vi "EtherNet_IP_CIP Demo.vi"() -> ()   [LabVIEW 2020, in "EtherNet_IP_CIP_Lib.lvlib"]
uses:
  EtherNet_IP_CIP_Lib.lvlib
panel:
  in  "CONTROL/TIMER/COUNTER":T1
  in  "REAL Array":sgl[](array[numeric])
  in  "DINT Array":u32[](array[numeric])
  in  "INT Array":u16[](array[numeric])
  in  "SINT Array":u8[](array[numeric])
  in  "BOOL Array":bool[](array[boolean])
  in  "BOOL Data":bool
  in  "Datatype":T2(ring)=enum."DINT"
  in  "Tag Name":string="EIPTXT01"
  in  "EtherNet/IP Device Address":string="192.168.1.214"
  out "REAL Array":sgl[](array[numeric])
  out "DINT Array":u32[](array[numeric]) format="%x"
  out "INT Array":u16[](array[numeric])
  out "SINT Array":u8[](array[numeric])
  out "CONTROL/TIMER/COUNTER":T1
  out "Datatype":T2(ring)
  out "BOOL Array":bool[](array[boolean])
  out "BOOL":bool
  out "Status":T3(ring)
  in  "Enter Tag Name":string="EIPTXT01"
  in  "No of Elements":u8
  out "Data Error":bool
  out "ms for Each Scan":u32
  out "error out":errorcluster
  in  "Exit":bool
  # "Write tag"
  # "Read Tag"
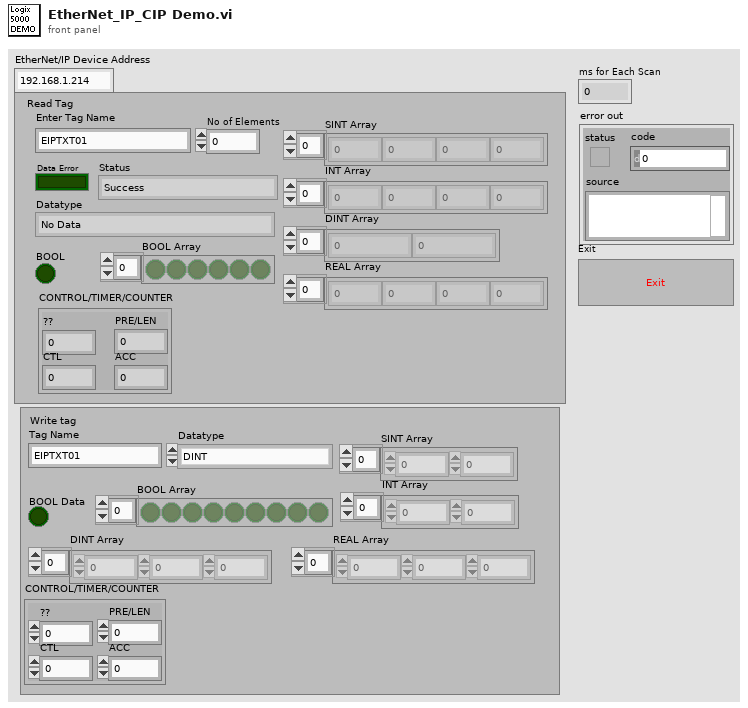
[diagram p1: front panel]
types:
  T1 = cluster{"??":u16, "CTL":u32, "PRE/LEN":u32, "ACC":u32}
  T2 = enum16{"No Data", "BOOL", "BIT Array", "SINT", "INT", "DINT", "REAL", "TIMER/CONTROL/COUNTER"}
  T3 = enum16{"Success", "Unknown Error", "Bad Symbolic Representation", "Item Not Found", "Partial Read", "Error Processing Attribute", "Incorrect/Insufficient Param", "Insufficient Attribute", "Bad Symbolic Length", "Out Of Bound", "Type Mismatch", "Offset Out Of Bound"}
  T4 = cluster{"TCP Connection":refnum<k5>, "Session":u8[], "EtherNet/IP Device Address":string}
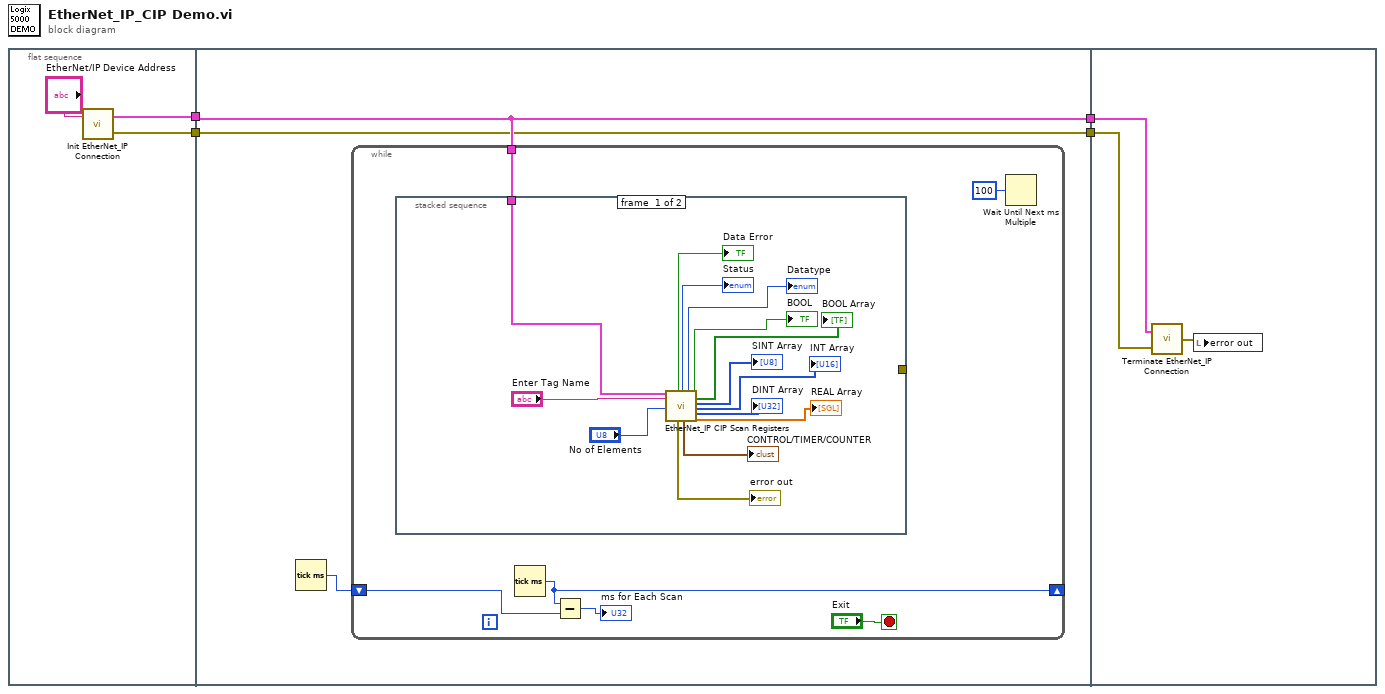
[diagram p0: block diagram]
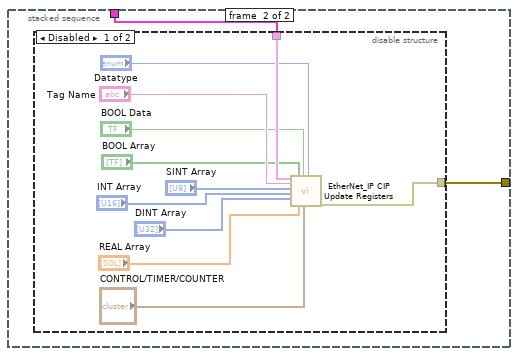
[diagram p2: hidden frame]
diagram:
  n1 = flat-sequence {
    tunnel: [w6] -> w4
    tunnel: [w5] -> w3
    tunnel: w4 -> [w10]
    tunnel: w3 -> [w8]
    tunnel: [w10] -> w2
    tunnel: [w8] -> w1
    tunnel: w2 -> [w46]
    tunnel: w1 -> [w45]
    frame #0 {
      n2 = call "Init EtherNet_IP Connection.vi"("EtherNet/IP Device Address"="EtherNet/IP Device Address") -> ("error out"=w5:errorcluster, "Connection Cluster"=w6:T4)  [unwired: 1 in]
    }
    frame #1 {
      n3 = Tick Count (ms)() -> (millisecond timer value=w9:u32)
      n4 = while {
        tunnel: w10 -> [w12]
        shift-right: [w15] -> _
        shift-left: w9 -> [w14]
        stop <- "Exit" stop-if-true
        n5 = stacked-sequence {
          tunnel: w12 -> [w29 w31]
          tunnel: [_ w32] -> _
          frame #0 {
            n6 = call "EtherNet_IP CIP Scan Registers.vi"("Connection Cluster"=w29, "Tag"="Enter Tag Name", "No of Elements"="No of Elements") -> ("Data Error"=→"Data Error":bool, "error out"=→"error out":errorcluster, "Status"=→"Status":T3, "CONTROL/TIMER/COUNTER"=→"CONTROL/TIMER/COUNTER":T1, "Datatype"=→"Datatype":T2, "BOOL"=→"BOOL":bool, "BOOL Array"=→"BOOL Array":bool[], "SINT Array"=→"SINT Array":u8[], "INT Array"=→"INT Array":u16[], "DINT Array"=→"DINT Array":u32[], "REAL Array"=→"REAL Array":sgl[])  [unwired: 5 in, 1 out]
          }
          frame #1 {
            n7 = disable-structure shown="Disabled" {
              disable-tunnel: [w42 _] -> w32
              disable-tunnel: w31 -> [w41 _]
              frame Disabled {
                n8 = call "EtherNet_IP CIP Update Registers.vi"("Connection Cluster"=w41, "Tag"="Tag Name", "SINT Array"="SINT Array", "INT Array"="INT Array", "DINT Array"="DINT Array", "BOOL Array"="BOOL Array", "REAL Array"="REAL Array", "BOOL"="BOOL Data", "CONTROL/TIMER/COUNTER"="CONTROL/TIMER/COUNTER", "Datatype"="Datatype") -> ("error out"=w42:errorcluster)  [unwired: 7 in, 2 out]
              }
              frame Enabled {
              }
            }
          }
        }
        n9 = Tick Count (ms)() -> (millisecond timer value=w15:u32)
        n10 = Subtract(x=w15, y=w14) -> (x-y=→"ms for Each Scan":u32)
        n11 = Wait Until Next ms Multiple(millisecond multiple=u32 100) -> ()  [unwired: 1 out]
      }
    }
    frame #2 {
      n12 = call "Terminate EtherNet_IP Connection.vi"("error in"=w45, "Connection Cluster"=w46) -> ("error out"=w44:errorcluster)
      n13 = local write "error out"(w44) -> ()
    }
  }
